vi "queueReaderTest.vi"() -> ()   [LabVIEW 2013]
uses:
  control/payloadData.ctl
  Global/GlobalStop.vi
panel:
  in  "ip/name":bool=TRUE
  out "cmd":string
  out "WatchDog":i32
  out "dataGramCount":i32
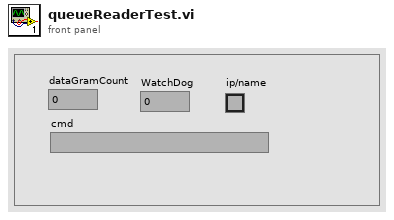
[diagram p1: front panel]
types:
  T1 = typedef "payloadData.ctl" = cluster{"Version":u32, "dataGramCount":i32, "cmd":string, "VariantData":variant}
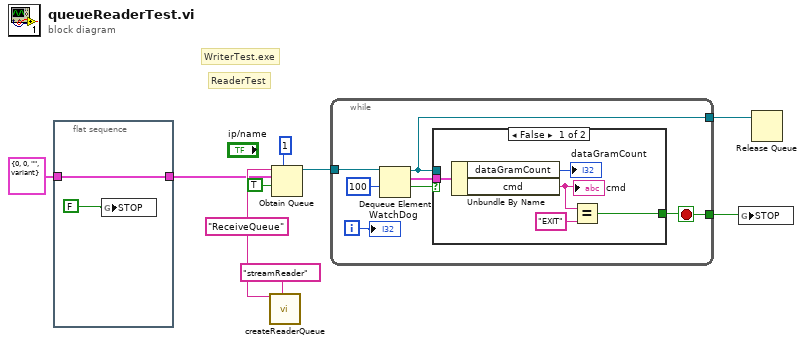
[diagram p0: block diagram]
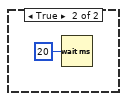
[diagram p2: hidden frame]
diagram:
  w9 = "ReceiveQueue"
  # "ReaderTest"
  # "WriterTest.exe"
  n1 = flat-sequence {
    tunnel: T1 {"Version"=0, "dataGramCount"=0, "cmd"="", "VariantData"=variant} ("Data") -> [w11]
    tunnel: [w11] -> w1
    frame #0 {
      n2 = global write "GlobalStop.vi" "STOP"(FALSE ("STOP")) -> ()
    }
  }
  n3 = call "createReaderQueue.vi"("QueueName"=w9, "ReaderEndPointName"="streamReader") -> ()  [unwired: 17 in, 1 out]
  n4 = Obtain Queue(max queue size (-1, unlimited)=1, name (unnamed)=w9, element data type=w1, create if not found? (T)=TRUE) -> (queue out=w8:refnum<queue>)  [unwired: 1 in, 2 out]
  n5 = while {
    tunnel: w8 -> [w18]
    tunnel: [w13] -> w5
    tunnel: [w12] -> w3
    i -> [w14]
    stop <- w12 stop-if-true
    n6 = Dequeue Element(queue=w18, timeout in ms (-1)=100) -> (queue out=w13:refnum<queue>, element=w15:T1, timed out?=w16:bool)  [unwired: 1 in, 1 out]
    n7 = case shown="False" w16 {
      tunnel: w13 -> [_ _]
      tunnel: w15 -> [w23 _]
      tunnel: [w19 _] -> w12
      frame False {
        n8 = Unbundle By Name(w23) -> ("dataGramCount"=→"dataGramCount":i32, "cmd"=w21:string)
        "cmd" <- w21
        n9 = Equal?(x=w21, y="EXIT") -> (x = y?=w19:bool)
      }
      frame True {
        n10 = Wait (ms)(milliseconds to wait=u32 20) -> ()  [unwired: 1 out]
      }
    }
    "WatchDog" <- w14
  }
  n11 = global write "GlobalStop.vi" "STOP"(w3) -> ()
  n12 = Release Queue(queue=w5) -> ()  [unwired: 2 in, 3 out]
